vi "Hang Immediate with Deadband.vi"(0 "Deploy?":bool, 1 "Description":string, 5 "Hang?":bool, 7 "Operation":T1, 9 "Rachet Engaged?":bool, 11 "Command Info In":T2, 12 "Deploy Color Wheel":bool) -> (15 "Command Info Out":T2)   [LabVIEW 2019]
doc: "This template includes code for deadband comparision to avoid excessive command scheduling. It is particularly useful for joystick-driven commands.\n\nBe sure to right-click and select New from Template and save with a new command name."
uses:
  <vilib>/Rock Robotics/WPI/Framework/Command Status Info.ctl
  <vilib>/Rock Robotics/WPI/Framework/Completion Status.ctl
  <vilib>/Rock Robotics/WPI/Framework/Completion Notifier.ctl
  Implementation/Hang Operations.ctl
  Implementation/Hang Setpoints.ctl
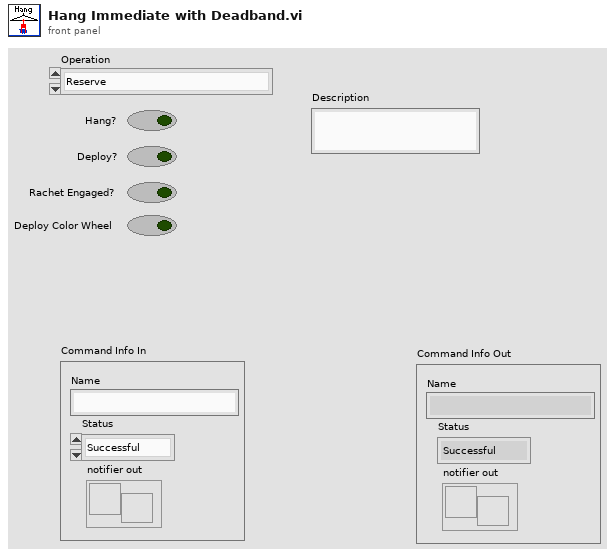
[diagram p1: front panel]
types:
  T1 = typedef "Hang Operations.ctl" = enum16{"Reserve", "Read Current", "Immediate", "Latch", "Un-Latch", "Color Wheel"}
  T2 = typedef "Command Status Info.ctl" = cluster{"Name":string, "Status":T3, "notifier out":T4}
  T3 = typedef "Completion Status.ctl" = enum16{"Successful", "Aborted", "Incomplete"}
  T4 = typedef "Completion Notifier.ctl" = refnum<notifier>
  T5 = typedef "Hang Setpoints.ctl" = cluster{"Operation":T1, "Rachet Engaged?":bool, "Deploy?":bool, "Hang?":bool, "Deploy Color Wheel":bool}
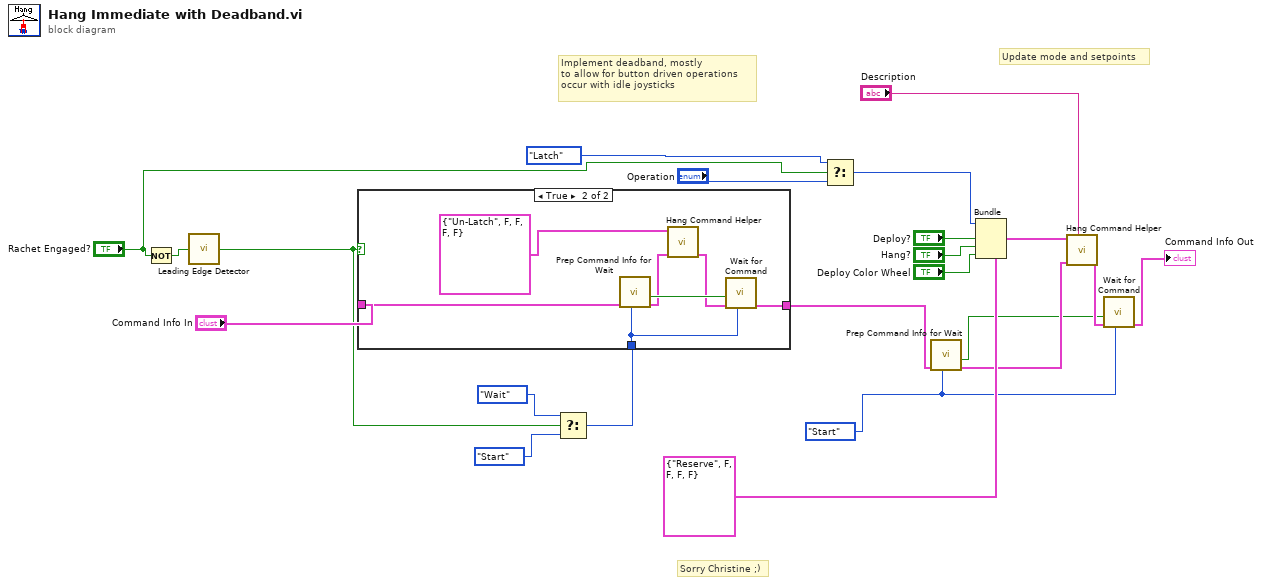
[diagram p0: block diagram]
diagram:
  w1 = enum16{"Start", "Wait"}."Start" ("Synchronication")
  # "Sorry Christine ;)"
  # "Implement deadband, mostly\nto allow for button driven operations\noccur with idle joysticks"
  # "Update mode and setpoints"
  n1 = Not(x="Rachet Engaged?") -> (.not. x?=w6:bool)
  n2 = call "Leading Edge Detector.vi"("Boolean"=w6) -> ("Out"=w7:bool)
  n3 = Select(t=enum16{"Start", "Wait"}."Wait" ("Synchronication"), s=w7, f=enum16{"Start", "Wait"}."Start" ("Synchronication")) -> (s? t:f=w8:enum16{"Start", "Wait"})
  n4 = case shown="True" w7 {
    tunnel: "Command Info In" -> [w23 w27]
    tunnel: [w23 w26] -> w12
    tunnel: w8 -> [_ w25]
    frame False {
    }
    frame True {
      n5 = call <vilib>:"Prep Command Info for Wait.vi"("Synchronication"=w25, "Command Info"=w27) -> ("Command Info"=w29:T2, "Allocated"=w30:bool)  [unwired: 8 in]
      n6 = call "Hang Command Helper.vi"("Command Info In"=w29, "SubSystem Data"=T5 {"Operation"=enum."Un-Latch", "Rachet Engaged?"=FALSE, "Deploy?"=FALSE, "Hang?"=FALSE, "Deploy Color Wheel"=FALSE}) -> ("Command Info Out"=w28:T2)  [unwired: 7 in, 2 out]
      n7 = call <vilib>:"Wait for Command.vi"("Synchronication"=w25, "Command Info in"=w28, "Allocated"=w30) -> ("Command Info out"=w26:T2)  [unwired: 8 in]
    }
  }
  n8 = Select(t=Hang_Operations."Latch" ("Operation"), s="Rachet Engaged?", f="Operation") -> (s? t:f=w2:T1)
  n9 = call <vilib>:"Prep Command Info for Wait.vi"("Synchronication"=w1, "Command Info"=w12) -> ("Command Info"=w15:T2, "Allocated"=w13:bool)  [unwired: 8 in]
  n10 = Bundle(cluster=T5 {"Operation"=enum."Reserve", "Rachet Engaged?"=FALSE, "Deploy?"=FALSE, "Hang?"=FALSE, "Deploy Color Wheel"=FALSE} ("SubSystem Data"), "Operation"=w2, "Deploy?"="Deploy?", "Hang?"="Hang?", "Deploy Color Wheel"="Deploy Color Wheel") -> (w20:T5)  [unwired: 1 in]
  n11 = call "Hang Command Helper.vi"("Description"="Description", "Command Info In"=w15, "SubSystem Data"=w20) -> ("Command Info Out"=w14:T2)  [unwired: 6 in, 2 out]
  n12 = call <vilib>:"Wait for Command.vi"("Synchronication"=w1, "Command Info in"=w14, "Allocated"=w13) -> ("Command Info out"=→"Command Info Out":T2)  [unwired: 8 in]
